vi "Local_Read_INI_Sub_VI_StateMachine.vi"(11 "Config File Path":path) -> (0 "output cluster":T1)   [LabVIEW 2017]
uses:
  <vilib>/Utility/config.llb/Read Key (I32).vi
  <vilib>/Utility/config.llb/Read Key (String).vi
  <vilib>/Utility/config.llb/Read Key (Path).vi
  <vilib>/Utility/config.llb/NI_LVConfig.lvlib
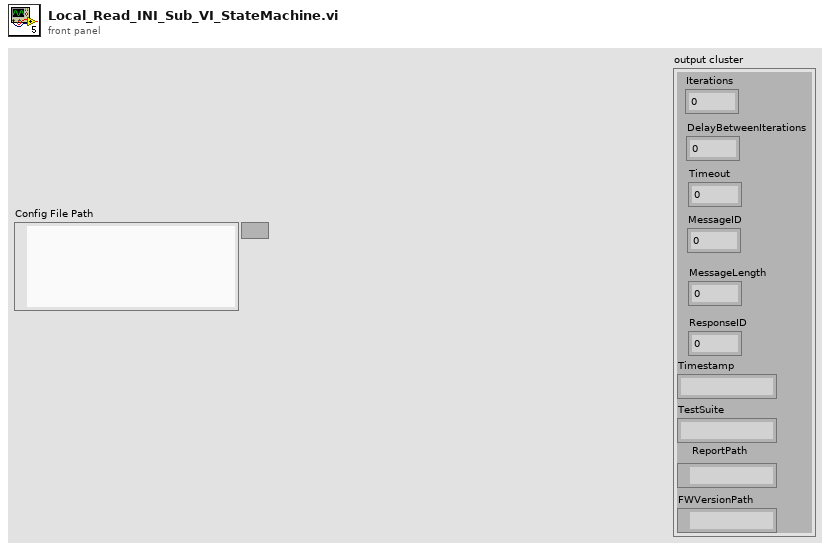
[diagram p1: front panel]
types:
  T1 = cluster{"Iterations":u64, "DelayBetweenIterations":u32, "Timeout":u32, "MessageID":i32, "MessageLength":i32, "ResponseID":i32, "Timestamp":string, "TestSuite":string, "ReportPath":path, "FWVersionPath":path}
  T2 = typedef "NI_LVConfig.lvlib/Config Data RefNum.ctl" = refnum<k1>
  T3 = cluster{u64, u32, u32, i32, i32, i32, "value":string, "value":string, "value":path, path}
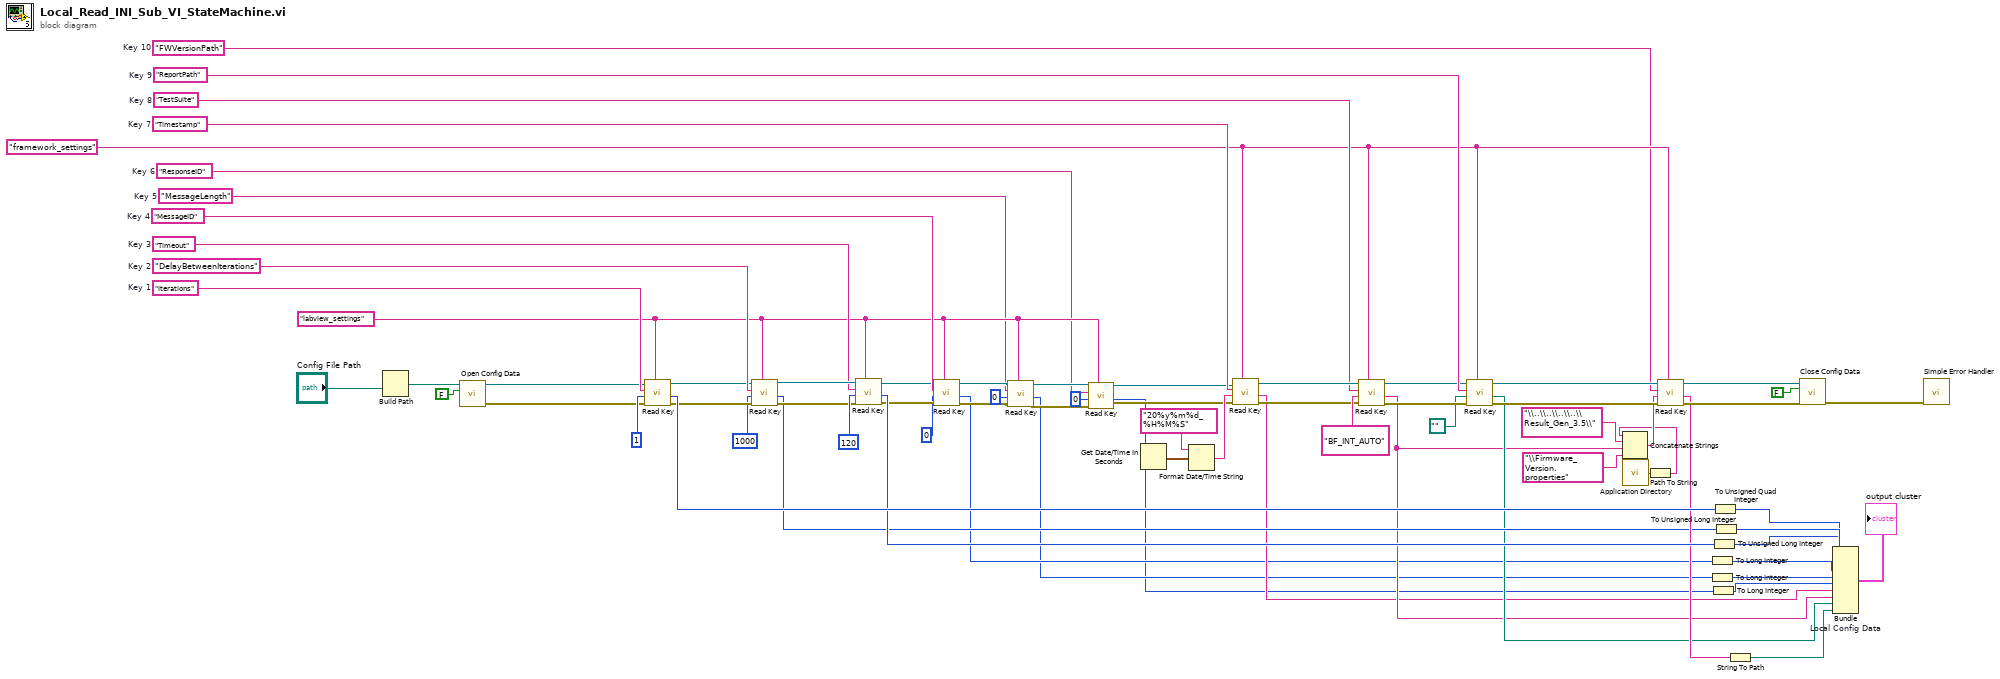
[diagram p0: block diagram]
diagram:
  w4 = "ResponseID"  # Key 6
  w5 = "MessageLength"  # Key 5
  w26 = "MessageID"  # Key 4
  w36 = "FWVersionPath"  # Key 10
  w48 = "Timestamp"  # Key 7
  w43 = "TestSuite"  # Key 8
  w49 = "Timeout"  # Key 3
  w58 = "ReportPath"  # Key 9
  w63 = "DelayBetweenIterations"  # Key 2
  w65 = "Iterations"  # Key 1
  w37 = "framework_settings" ("section")
  w25 = "labview_settings" ("section")
  n1 = Build Path(name or relative path="Config File Path") -> (appended path=w67:path)  [unwired: 1 in]
  n2 = call <vilib>:"Open Config Data.vi"("create file if necessary (T)"=FALSE ("create file if necessary? (T)"), "configuration file path"=w67) -> ("error out"=w29:errorcluster, "refnum"=w28:T2)  [unwired: 7 in, 1 out]
  n3 = call-poly <vilib>:"Read Key.vi"("section"=w25, "error in (no error)"=w29, "default value"=1, "key"=w65, "refnum"=w28) -> ("error out"=w61:errorcluster, "value"=w64:i32, "refnum out"=w62:T2)  [unwired: 4 out]
  n4 = call-poly <vilib>:"Read Key.vi"("section"=w25, "error in (no error)"=w61, "default value"=1000, "key"=w63, "refnum"=w62) -> ("error out"=w56:errorcluster, "value"=w27:i32, "refnum out"=w55:T2)  [unwired: 4 out]
  n5 = call-poly <vilib>:"Read Key.vi"("section"=w25, "error in (no error)"=w56, "default value"=120, "key"=w49, "refnum"=w55) -> ("error out"=w20:errorcluster, "value"=w53:i32, "refnum out"=w24:T2)  [unwired: 4 out]
  n6 = call-poly <vilib>:"Read Key.vi"("section"=w25, "error in (no error)"=w20, "default value"=0, "key"=w26, "refnum"=w24) -> ("error out"=w18:errorcluster, "value"=w12:i32, "refnum out"=w23:T2)  [unwired: 4 out]
  n7 = call-poly <vilib>:"Read Key.vi"("section"=w25, "error in (no error)"=w18, "default value"=0, "key"=w5, "refnum"=w23) -> ("error out"=w19:errorcluster, "value"=w8:i32, "refnum out"=w22:T2)  [unwired: 4 out]
  n8 = call-poly <vilib>:"Read Key.vi"("section"=w25, "error in (no error)"=w19, "default value"=0, "key"=w4, "refnum"=w22) -> ("error out"=w17:errorcluster, "value"=w7:i32, "refnum out"=w21:T2)  [unwired: 4 out]
  n9 = Get Date/Time In Seconds() -> (seconds since 1Jan1904=w50:timestamp)
  n10 = Format Date/Time String(time format string (%c)="20%y%m%d_%H%M%S", seconds (now)=w50) -> (date/time string=w51:string)  [unwired: 1 out]
  n11 = call-poly <vilib>:"Read Key.vi"("section"=w37, "error in (no error)"=w17, "default value"=w51, "key"=w48, "refnum"=w21) -> ("error out"=w45:errorcluster, "value"=w13:string, "refnum out"=w46:T2)  [unwired: 1 in, 3 out]
  n12 = call-poly <vilib>:"Read Key.vi"("section"=w37, "error in (no error)"=w45, "default value"="BF_INT_AUTO", "key"=w43, "refnum"=w46) -> ("error out"=w44:errorcluster, "value"=w14:string, "refnum out"=w47:T2)  [unwired: 1 in, 3 out]
  n13 = call-poly <vilib>:"Read Key.vi"("section"=w37, "error in (no error)"=w44, "default value"=path "", "key"=w58, "refnum"=w47) -> ("error out"=w38:errorcluster, "value"=w15:path, "refnum out"=w41:T2)  [unwired: 1 in, 3 out]
  n14 = call <vilib>:"Application Directory.vi"() -> ("Application Directory"=w32:path)
  n15 = Path To String(path=w32) -> (string=w31:string)
  n16 = Concatenate Strings(w31, "\\..\\..\\..\\..\\Result_Gen_3.5\\" ("default value"), w14, "\\Firmware_Version.properties" ("default value")) -> (w35:string)
  n17 = call-poly <vilib>:"Read Key.vi"("section"=w37, "error in (no error)"=w38, "default value"=w35, "key"=w36, "refnum"=w41) -> ("error out"=w39:errorcluster, "value"=w30:string, "refnum out"=w40:T2)  [unwired: 1 in, 3 out]
  n18 = To Long Integer(number=w12) -> (32bit integer=w11:i32)
  n19 = To Long Integer(number=w8) -> (32bit integer=w10:i32)
  n20 = To Long Integer(number=w7) -> (32bit integer=w9:i32)
  n21 = To Unsigned Long Integer(number=w53) -> (unsigned 32bit integer=w72:u32)
  n22 = To Unsigned Quad Integer(1:w64) -> (0:w71:u64)
  n23 = To Unsigned Long Integer(number=w27) -> (unsigned 32bit integer=w73:u32)
  n24 = String To Path(string=w30) -> (path=w16:path)
  n25 = call <vilib>:"Close Config Data.vi"("error in (no error)"=w39, "write file if changed (T)"=FALSE ("write configuration file? (T)"), "refnum"=w40) -> ("error out"=w68:errorcluster)  [unwired: 8 out]
  n26 = Bundle "Local Config Data"(w71, w73, w72, w11, w10, w9, "value"=w13, "value"=w14, "value"=w15, w16) -> (→"output cluster":T3)  [unwired: 1 in]
  n27 = call <vilib>:"Simple Error Handler.vi"("error in (no error)"=w68) -> ()  [unwired: 1 in, 8 out]
